vi "construct.vi"(8 "error in (no error)":errorcluster, 9 "configuration name":string, 10 "load config file?":bool=TRUE, 11 "GenericPlugin in":refnum<class "StimulatorAK101022TCP.lvclass">) -> (0 "error out":errorcluster, 3 "GenericPlugin out":refnum<class "StimulatorAK101022TCP.lvclass">)   [LabVIEW 2010, in "StimulatorAK101022TCP.lvclass"]
uses:
  StimulatorAK101022TCP.lvclass
  StimulatorDL090503Scaffold/StimulatorDL090503Scaffold/StimulatorDL090503Scaffold.lvclass
  StimulatorAK101022TCP.lvclass/StimulatorAK101022TCP.ctl
  StringGenerator/GenericStringGenerator/GenericStringGenerator/GenericStringGenerator.lvclass
  common/classes/GenericComponent/GenericComponent/GenericComponent.lvclass
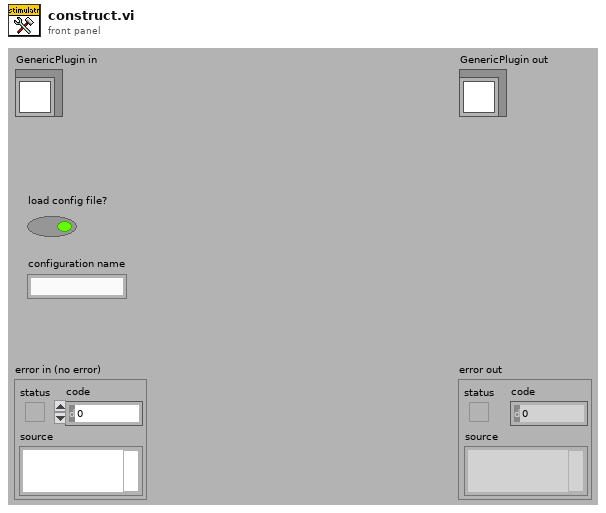
[diagram p1: front panel]
types:
  T1 = typedef "plugin_specification.ctl" = cluster{"class path":string, "configuration":string, "label":string, "settings name":string}
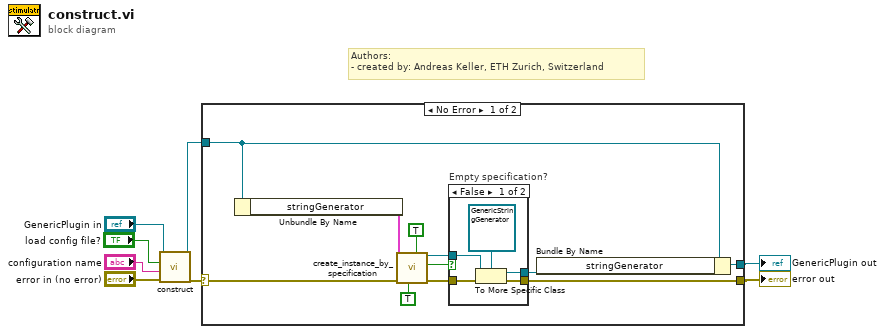
[diagram p0: block diagram]
diagram:
  # "Authors: \n- created by: Andreas Keller, ETH Zurich, Switzerland"
  n1 = call-parent "construct.vi"("error in (no error)"="error in (no error)", "configuration name"="configuration name", "load config file?"="load config file?", "GenericPlugin in"="GenericPlugin in") -> ("error out"=w4:errorcluster, "GenericPlugin out"=w1:refnum<class "StimulatorAK101022TCP.lvclass">)  [unwired: 6 in]
  n2 = case shown="No Error" w4 {
    selector: w4 -> [w15 w26]
    tunnel: [w14 w26] -> w3
    tunnel: [w13 w27] -> w2
    tunnel: w1 -> [w11 w27]
    frame No Error {
      n3 = Unbundle By Name(w11) -> ("stringGenerator"=w19:T1)
      n4 = call "create_instance_by_specification.vi"("be tolerant against empty specification?"=TRUE, "call constructor?"=TRUE, "error in (no error)"=w15, "component specification"=w19) -> ("error out"=w17:errorcluster, "empty specification!"=w9:bool, "GenericPlugin out"=w16:refnum<class "GenericComponent.lvclass">)  [unwired: 5 in]
      n5 = case "Empty specification?" shown="False" w9 {
        tunnel: w17 -> [w24 w25]
        tunnel: w16 -> [w23 _]
        tunnel: [w22 w25] -> w14
        tunnel: [w20 _] -> w12
        frame False {
          n6 = To More Specific Class(target class=refnum<class "GenericStringGenerator.lvclass"> refnum ("GenericStringGenerator.lvclass"), reference=w23, error in=w24) -> (specific class reference=w20:refnum<class "GenericStringGenerator.lvclass">, error out=w22:errorcluster)
        }
        frame True {
        }
      }
      n7 = Bundle By Name(cluster=w11, "stringGenerator"=w12) -> (w13:refnum<class "StimulatorAK101022TCP.lvclass">)
    }
    frame Error {
    }
  }
  "error out" <- w3
  "GenericPlugin out" <- w2
